vi "Setup file input channels.vi"(8 "error in":errorcluster, 9 "Sampling data":T1={"Channels"=[], "Sampling freq"=0, "Output freq"=0, "Update freq"=0, "Steps per rev"=0, "Counts per rev"=0, "Amplifier"="", "Motor driver"="", "Step bit"=0, "Max speed"=0.0, "Max accel"=0.0, "Pos gain"=0.0, "Vel gain"=0.0, "counter"="Dev1/ctr0"} {"Channels"."Hi cutoff" items=["500"=500.0, "1k"=1000.0, "5k"=5000.0, "10k"=10000.0, "20k"=20000.0]; "Channels"."Lo cutoff" items=["0.1"=0.1, "1"=1.0, "10"=10.0, "100"=100.0, "300"=300.0]; "Channels"."Gain" items=["x100"=100, "x1000"=1000, "x10000"=10000]}, 11 "file ref in":T3 format="%.0x") -> (0 "error out":errorcluster, 1 "Sampling data out":T1={"Channels"=[], "Sampling freq"=0, "Output freq"=0, "Update freq"=0, "Steps per rev"=0, "Counts per rev"=0, "Amplifier"="", "Motor driver"="", "Step bit"=0, "Max speed"=0.0, "Max accel"=0.0, "Pos gain"=0.0, "Vel gain"=0.0, "counter"="Dev1/ctr0"} {"Channels"."Hi cutoff" items=["500"=500.0, "1k"=1000.0, "5k"=5000.0, "10k"=10000.0, "20k"=20000.0]; "Channels"."Lo cutoff" items=["0.1"=0.1, "1"=1.0, "10"=10.0, "100"=100.0, "300"=300.0]; "Channels"."Gain" items=["x100"=100, "x1000"=1000, "x10000"=10000]}, 2 "dset ref":i32, 3 "file ref out":T3 format="%.0x", 4 "encoder dset":i32)   [LabVIEW 2012]
uses:
  <vilib>/addons/h5labview2/base/hid_t.ctl
  Sampling info.ctl
  Channel.ctl
  Create HDF5 chunked dataset (1D).vi
  Create HDF5 chunked dataset (2D).vi
  <vilib>/addons/h5labview2/base/H5Equery.vi
  <vilib>/addons/h5labview2/attrib/H5Awrite.llb/H5Awrite.xnode
  <vilib>/addons/h5labview2/group/H5G.lvlib
  <vilib>/addons/h5labview2/h5labview32.dll
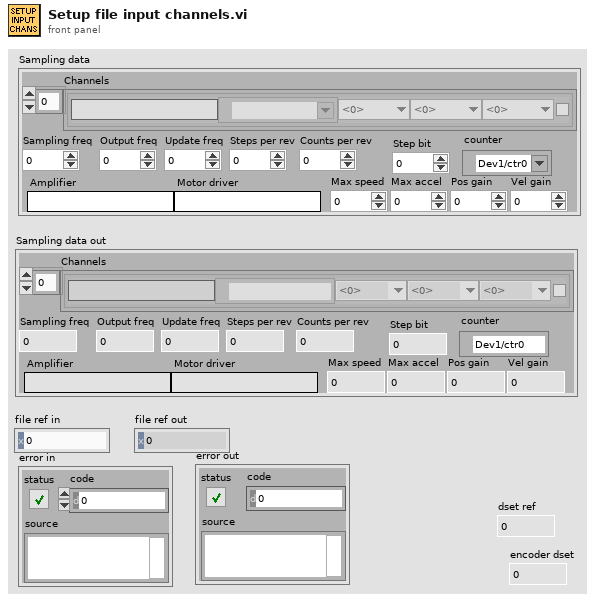
[diagram p1: front panel]
types:
  T1 = typedef "Sampling info.ctl" = cluster{"Channels":T2[], "Sampling freq":i32, "Output freq":i32, "Update freq":i32, "Steps per rev":i32, "Counts per rev":i32, "Amplifier":string, "Motor driver":string, "Step bit":u8, "Max speed":dbl, "Max accel":dbl, "Pos gain":dbl, "Vel gain":dbl, "counter":tag}
  T2 = typedef "Channel.ctl" = cluster{"Name":string, "Chan":tag, "Gain":u16, "Lo cutoff":dbl, "Hi cutoff":dbl, "Notch":bool}
  T3 = typedef "hid_t.ctl" = i32
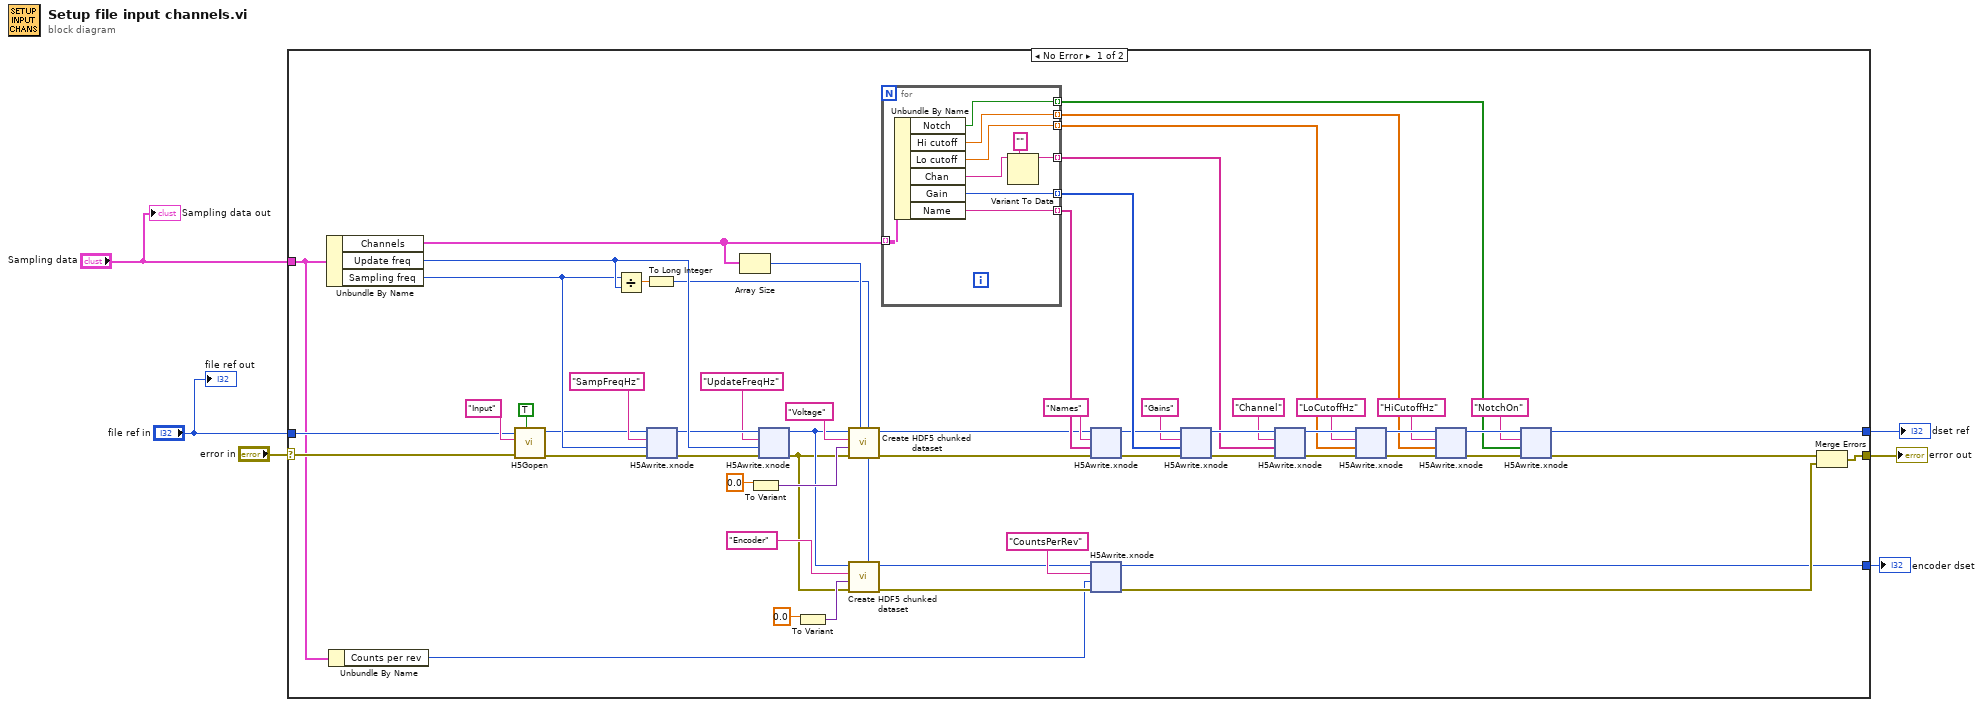
[diagram p0: block diagram]
diagram:
  n1 = case shown="No Error" "error in" {
    selector: "error in" -> [w24 w227]
    tunnel: [w64 _] -> w6
    tunnel: [w10 w227] -> w5
    tunnel: "file ref in" -> [w23 _]
    tunnel: "Sampling data" -> [w12 _]
    tunnel: [w7 _] -> w1
    frame No Error {
      n2 = Unbundle By Name(w12) -> ("Channels"=w47:T2[], "Update freq"=w43:i32, "Sampling freq"=w42:i32)
      n3 = Unbundle By Name(w12) -> ("Counts per rev"=w11:i32)
      n4 = call <vilib>:"H5Gopen.vi"("create? (F)"=TRUE, "error in (no error)"=w24, "name"="Input", "ref in"=w23) -> ("error out"=w29:errorcluster, "group out"=w30:T3)  [unwired: 3 in]
      n5 = Divide(x=w42, y=w43) -> (x/y=w44:dbl)
      n6 = To Long Integer(number=w44) -> (32bit integer=w16:i32)
      n7 = xnode "H5Awrite.xnode"("error in (no error)"=w29, "data"=w42, "attrib name"="SampFreqHz", "ref in"=w30) -> ("error out"=w34:errorcluster, "ref out"=w33:i32)  [unwired: 3 in, 1 out]
      n8 = Array Size(array=w47) -> (size(s)=w22:i32)
      n9 = To Variant(anything=0.0) -> (Variant=w25:variant)
      n10 = xnode "H5Awrite.xnode"("error in (no error)"=w34, "data"=w43, "attrib name"="UpdateFreqHz", "ref in"=w33) -> ("error out"=w17:errorcluster, "ref out"=w18:i32)  [unwired: 3 in, 1 out]
      n11 = To Variant(anything=0.0) -> (Variant=w21:variant)
      n12 = call-poly "Create HDF5 chunked dataset.vi"("block size"=w16, "number of channels"=w22, "error in (no error)"=w17, "data type"=w25, "name"="Voltage", "ref in"=w18) -> ("error out"=w38:errorcluster, "dset out"=w36:i32)  [unwired: 4 in]
      n13 = call-poly "Create HDF5 chunked dataset.vi"("block size"=w16, "error in (no error)"=w17, "data type"=w21, "name"="Encoder", "ref in"=w18) -> ("error out"=w13:errorcluster, "dset out"=w14:i32)  [unwired: 5 in]
      n14 = for {
        tunnel: w47 -> [w192] mode=indexing
        tunnel: [w191] -> w45 mode=indexing
        tunnel: [w190] -> w46 mode=indexing
        tunnel: [w187] -> w49 mode=indexing
        tunnel: [w186] -> w53 mode=indexing
        tunnel: [w185] -> w54 mode=indexing
        tunnel: [w184] -> w55 mode=indexing
        n15 = Unbundle By Name(w192) -> ("Notch"=w184:bool, "Hi cutoff"=w185:dbl, "Lo cutoff"=w186:dbl, "Chan"=w189:tag, "Gain"=w190:u16, "Name"=w191:string)
        n16 = Variant To Data(type="", Variant=w189) -> (data=w187:string)  [unwired: 1 in, 1 out]
      }
      n17 = xnode "H5Awrite.xnode"("error in (no error)"=w38, "data"=w45, "attrib name"="Names", "ref in"=w36) -> ("error out"=w41:errorcluster, "ref out"=w40:i32)  [unwired: 3 in, 1 out]
      n18 = xnode "H5Awrite.xnode"("error in (no error)"=w13, "data"=w11, "attrib name"="CountsPerRev", "ref in"=w14) -> ("error out"=w8:errorcluster, "ref out"=w7:i32)  [unwired: 3 in, 1 out]
      n19 = xnode "H5Awrite.xnode"("error in (no error)"=w41, "data"=w46, "attrib name"="Gains", "ref in"=w40) -> ("error out"=w57:errorcluster, "ref out"=w56:i32)  [unwired: 3 in, 1 out]
      n20 = xnode "H5Awrite.xnode"("error in (no error)"=w57, "data"=w49, "attrib name"="Channel", "ref in"=w56) -> ("error out"=w59:errorcluster, "ref out"=w58:i32)  [unwired: 3 in, 1 out]
      n21 = xnode "H5Awrite.xnode"("error in (no error)"=w59, "data"=w53, "attrib name"="LoCutoffHz", "ref in"=w58) -> ("error out"=w61:errorcluster, "ref out"=w60:i32)  [unwired: 3 in, 1 out]
      n22 = xnode "H5Awrite.xnode"("error in (no error)"=w61, "data"=w54, "attrib name"="HiCutoffHz", "ref in"=w60) -> ("error out"=w62:errorcluster, "ref out"=w63:i32)  [unwired: 3 in, 1 out]
      n23 = xnode "H5Awrite.xnode"("error in (no error)"=w62, "data"=w55, "attrib name"="NotchOn", "ref in"=w63) -> ("error out"=w9:errorcluster, "ref out"=w64:i32)  [unwired: 3 in, 1 out]
      n24 = Merge Errors(w9, w8) -> (w10:errorcluster)
    }
    frame Error {
    }
  }
  "dset ref" <- w6
  "error out" <- w5
  "encoder dset" <- w1
  "file ref out" <- "file ref in"
  "Sampling data out" <- "Sampling data"
